vi "EXFO.vi"() -> ()   [LabVIEW 2014]
panel:
  out "String":string
  out "Error Out":errorcluster
  out "Return Code":i32
  out "Python Error":string
  out "EXFO Output":string
  in  "Path":path
  in  "EXFO Python Script":string
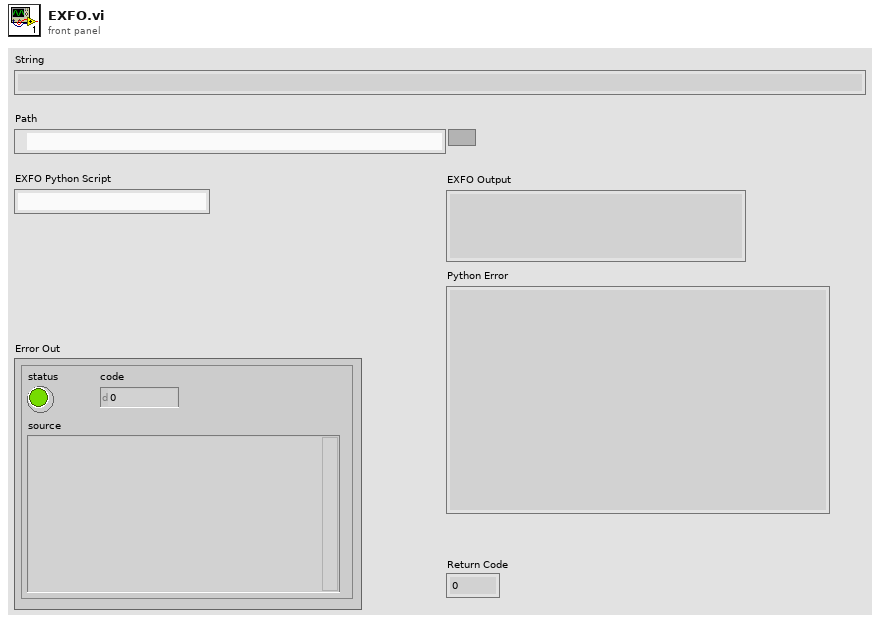
[diagram p1: front panel]
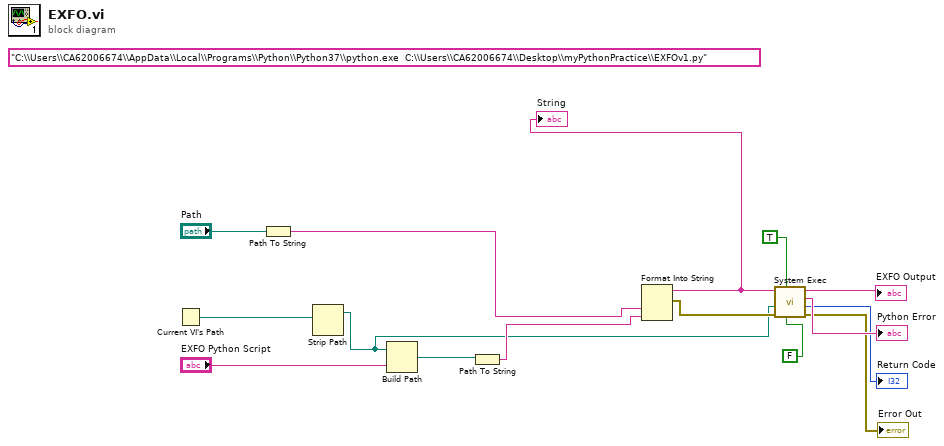
[diagram p0: block diagram]
diagram:
  (unwired) "C:\\Users\\CA62006674\\AppData\\Local\\Programs\\Python\\Python37\\python.exe  C:\\Users\\CA62006674\\Desktop\\myPythonPractice\\EXFOv1.py"
  n1 = Current VI's Path() -> (path=w15:path)
  n2 = Path To String(path="Path") -> (string=w5:string)
  n3 = Strip Path(path=w15) -> (stripped path=w1:path)  [unwired: 1 out]
  n4 = Build Path(base path=w1, name or relative path="EXFO Python Script") -> (appended path=w13:path)
  n5 = Path To String(path=w13) -> (string=w4:string)
  n6 = Format Into String(w5, w4) -> (resulting string=w3:string, error out=w11:errorcluster)  [unwired: 3 in]
  "String" <- w3
  n7 = call <vilib>:"System Exec.vi"("run minimized? (F)"=FALSE, "wait until completion? (T)"=TRUE, "error in (no error)"=w11, "working directory"=w1, "command line"=w3) -> ("error out"=→"Error Out":errorcluster, "return code"=→"Return Code":i32, "standard error"=→"Python Error":string, "standard output"=→"EXFO Output":string)  [unwired: 3 in]
